vi "DS402 Drive - Compare ECAT Vars.vi"(8 "Fehler (Eingang, kein Fehler)":errorcluster, 11 "I/O Vars In":T1[](array[typedef]) {"VS ref" format="%.0x"}) -> (0 "Fehler (Ausgang)":errorcluster, 3 "I/O Vars Out":T1[](array[typedef]) {"VS ref" format="%.0x"})   [LabVIEW 2016, in "Scan Engine Custom Device.lvlib"]
uses:
  Scan Engine Custom Device.lvlib
  Type Defs/DS402 Drive ECAT Slave IOV Cluster.ctl
  <vilib>/NI Veristand/Custom Device API/Custom Device Item Ref.ctl
  Type Defs/UDV Data Type.ctl
  Globals/Property Strings.vi
  <vilib>/NI Veristand/Custom Device API/Get Item Property (I32).vi
  Globals/Error Strings.vi
  <vilib>/NI Veristand/Custom Device API/Custom Device API.lvlib
  <vilib>/NI Veristand/Custom Device Tools/Custom Device Utility Library/Custom Device Utility Library.lvlib
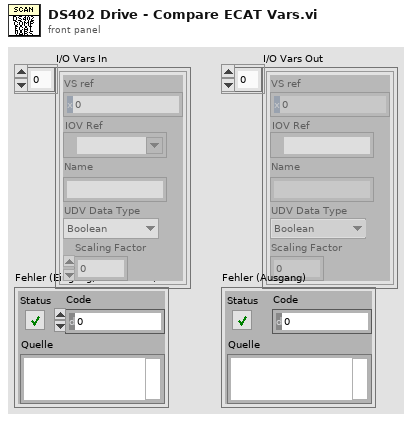
[diagram p1: front panel]
types:
  T1 = typedef "Scan Engine Custom Device.lvlib/DS402 Drive ECAT Slave IOV Cluster.ctl" = cluster{"VS ref":T2, "IOV Ref":refnum<k21>, "Name":string, "UDV Data Type":T3, "Scaling Factor":dbl}
  T2 = typedef "Custom Device API.lvlib/Custom Device Item Ref.ctl" = u64
  T3 = typedef "Scan Engine Custom Device.lvlib/UDV Data Type.ctl" = enum16{"Boolean", "Fixed Point", "Int8", "Int16", "Int32", "Int64", "U32 Bit Field", "UInt8", "UInt16", "UInt32", "UInt64", "Other"}
  T4 = typedef "Custom Device API.lvlib/Custom Device Item Info.ctl" = cluster{"Name":string, "Is Channel":bool, "GUID":string, "Is Waveform":bool}
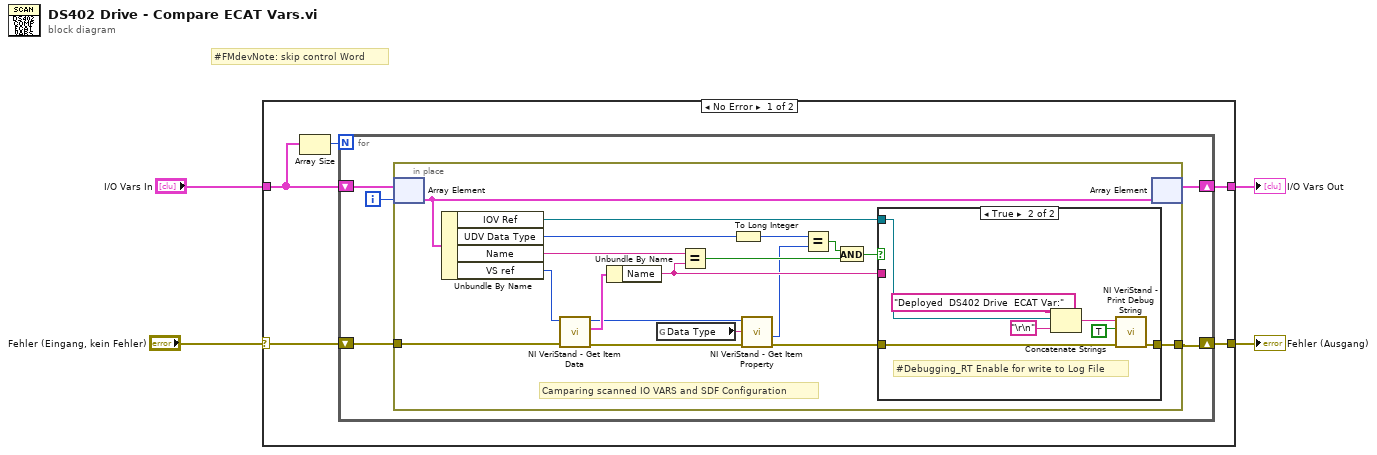
[diagram p0: block diagram]
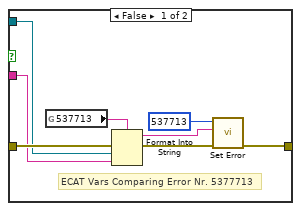
[diagram p2: hidden frame]
diagram:
  # "#FMdevNote: skip control Word"
  n1 = case shown="No Error" "Fehler (Eingang, kein Fehler)" {
    selector: "Fehler (Eingang, kein Fehler)" -> [w8 w49]
    tunnel: [w5 w48] -> w1
    tunnel: [w7 w49] -> w4
    tunnel: "I/O Vars In" -> [w6 w48]
    frame No Error {
      n2 = Array Size(array=w6) -> (size(s)=w9:i32)
      n3 = for {
        N: w9 -> [_]
        shift-right: [w12] -> w7
        shift-left: w8 -> [w13]
        shift-right: [w10] -> w5
        shift-left: w6 -> [w11]
        i -> [w14]
        n4 = in-place {
          in-place-border: w13 -> [w28]
          in-place-border: [w23] -> w12
          # "Camparing scanned IO VARS and SDF Configuration"
          n5 = in-place-array #1(w11, w14) -> (w18:T1)
          n6 = Unbundle By Name(w18) -> ("IOV Ref"=w21:refnum<k21>, "UDV Data Type"=w22:T3, "Name"=w17:string, "VS ref"=w19:T2)
          n7 = call <vilib>:"NI VeriStand - Get Item Data.vi"("error in (no error)"=w28, "Item Ref in"=w19) -> ("error out"=w31:errorcluster, "Item Info"=w32:T4, "Item Ref out"=w30:T2)  [unwired: 6 in, 1 out]
          n8 = Unbundle By Name(w32) -> ("Name"=w20:string)
          n9 = global read "Property Strings.vi" "Data Type"() -> (w29:string)
          n10 = Equal?(x=w17, y=w20) -> (x = y?=w26:bool)
          n11 = To Long Integer(number=w22) -> (32bit integer=w15:i32)
          n12 = call-poly <vilib>:"NI VeriStand - Get Item Property.vi"("error in (no error)"=w31, "Property Name"=w29, "Item Ref in"=w30) -> ("error out"=w24:errorcluster, "Value"=w16:i32)  [unwired: 5 in, 2 out]
          n13 = Equal?(x=w15, y=w16) -> (x = y?=w27:bool)
          n14 = And(x=w27, y=w26) -> (x .and. y?=w25:bool)
          n15 = case shown="True" w25 {
            tunnel: w24 -> [w36 w47]
            tunnel: [w35 w46] -> w23
            tunnel: w21 -> [w34 w42]
            tunnel: w20 -> [w33 _]
            frame False {
              # "ECAT Vars Comparing Error Nr. 5377713"
              n16 = global read "Error Strings.vi" "537713"() -> (w37:string)
              n17 = Format Into String(format string=w37, error in=w36, w34, w33) -> (resulting string=w39:string, error out=w38:errorcluster)  [unwired: 1 in]
              n18 = call "Set Error.vi"("error in (no error)"=w38, "Message"=w39, "Code"=537713 ("error code (0)")) -> ("error out"=w35:errorcluster)  [unwired: 8 in]
            }
            frame True {
              # "#Debugging_RT Enable for write to Log File"
              n19 = Concatenate Strings("Deployed  DS402 Drive  ECAT Var:", w42, "\r\n") -> (w45:string)
              n20 = call <vilib>:"NI VeriStand - Print Debug String.vi"("error in (no error)"=w47, "Add to log file? (T)"=TRUE, "Message"=w45) -> ("error out"=w46:errorcluster)  [unwired: 8 in]
            }
          }
          n21 = in-place-array #1(w18) -> (w10:T1[])  [unwired: 1 out]
        }
      }
    }
    frame Error {
    }
  }
  "I/O Vars Out" <- w1
  "Fehler (Ausgang)" <- w4
